vi "ContourFilledAuto2001.vi"   [LabVIEW 2013]
uses:
  ModeType.ctl
  <vilib>/Heliosphere Research LLC/Advanced Plotting Toolkit/api_plotting/ContourFilled_Automatic.vi
  <vilib>/Heliosphere Research LLC/Advanced Plotting Toolkit/Advanced Plotting Toolkit.lvlib
types:
  T1 = typedef "ModeType.ctl" = enum16{"Normal", "Expected Failure", "Skipped", "Broken"}
  T2 = typedef "Advanced Plotting Toolkit.lvlib/PlotID.ctl" = i32
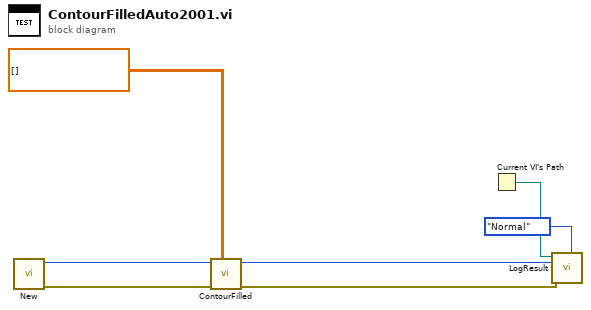
[diagram p0: block diagram]
diagram:
  n1 = call <vilib>:"New.vi"() -> ("error out"=w5:errorcluster, "Plot ID"=w6:T2)  [unwired: 10 in]
  n2 = call-poly <vilib>:"ContourFilled.vi"("Z Data"=dbl[][] [], "error in (no error)"=w5, "Plot ID"=w6) -> ("error out"=w3:errorcluster, "Plot ID Out"=w4:T2)  [unwired: 7 in]
  n3 = Current VI's Path() -> (path=w7:path)
  n4 = call "LogResult.vi"("Mode"=ModeType."Normal", "Test Result"=w3, "Test Artifact"=w4, "VI Path"=w7) -> ()  [unwired: 8 in]
